vi "3.0-Loop Super Heart Beat.vi"() -> (0 "Super Heart Beat":T1)   [LabVIEW 2010]
uses:
  4-High Neurons/4.0-Super Heart Beat.ctl
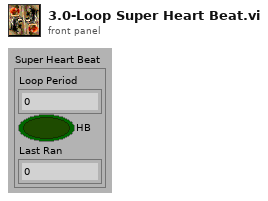
[diagram p1: front panel]
types:
  T1 = typedef "4.0-Super Heart Beat.ctl" = cluster{"Loop Period":u32, "HB":bool, "Last Ran":u32}
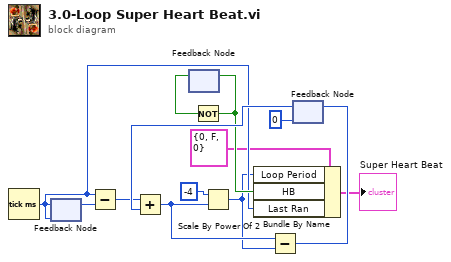
[diagram p0: block diagram]
diagram:
  n1 = Tick Count (ms)() -> (millisecond timer value=w4:u32)
  n2 = feedback #1(w4) -> (w13:u32)
  n3 = feedback-in #1(w4) -> ()
  n4 = Subtract(x=w4, y=w13) -> (x-y=w6:u32)
  n5 = feedback #2() -> (w8:bool)  [unwired: 1 in]
  n6 = Not(x=w8) -> (.not. x?=w7:bool)
  n7 = feedback-in #2(w7) -> ()
  n8 = feedback #3(u32 0) -> (w12:u32)
  n9 = Add(x=w6, y=w12) -> (x+y=w11:u32)
  n10 = Scale By Power Of 2(n=-4, x=w11) -> (x*2^n=w3:u32)
  n11 = Bundle By Name(cluster=T1 {"Loop Period"=0, "HB"=FALSE, "Last Ran"=0} ("Loop Update Cluster"), "Loop Period"=w3, "HB"=w7, "Last Ran"=w4) -> (→"Super Heart Beat":T1)
  n12 = Subtract(x=w11, y=w3) -> (x-y=w10:u32)
  n13 = feedback-in #3(w10) -> ()
